vi "SetArrayDevParams.vi"(0 "Interface.lvclass":refnum<class "Interface.lvclass">, 1 "DescKword":string, 5 "Save":bool, 9 "Experiment.lvclass":refnum<class "Experiment.lvclass">, 11 "error in":errorcluster, 12 "ArrayFuncName":string) -> (3 "DataFileRef":refnum<file>, 4 "Interf.lvclass Out":refnum<class "Interface.lvclass">, 6 "DataFileName":path, 10 "Exp.lvclass Out":refnum<class "Experiment.lvclass">, 14 "Scan list":string[](array[string]), 15 "error out":errorcluster)   [LabVIEW 2019, in "Interface.lvclass"]
doc: "Ce Vi prend les données d'acquisition et les formatte en tableau de \"string\" pour ensuite les sauvegarder sous le format .txt"
uses:
  Interface.lvclass
  Experiment Class/Experiment.lvclass
  Interface.lvclass/Interface.ctl
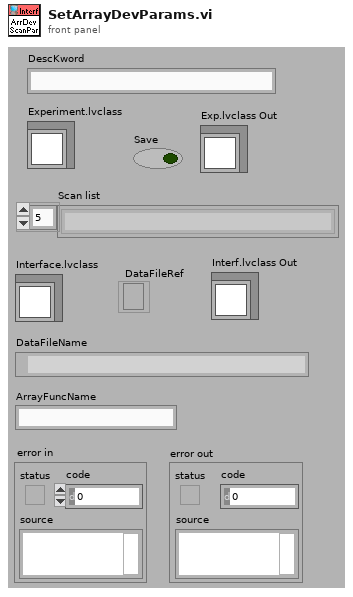
[diagram p1: front panel]
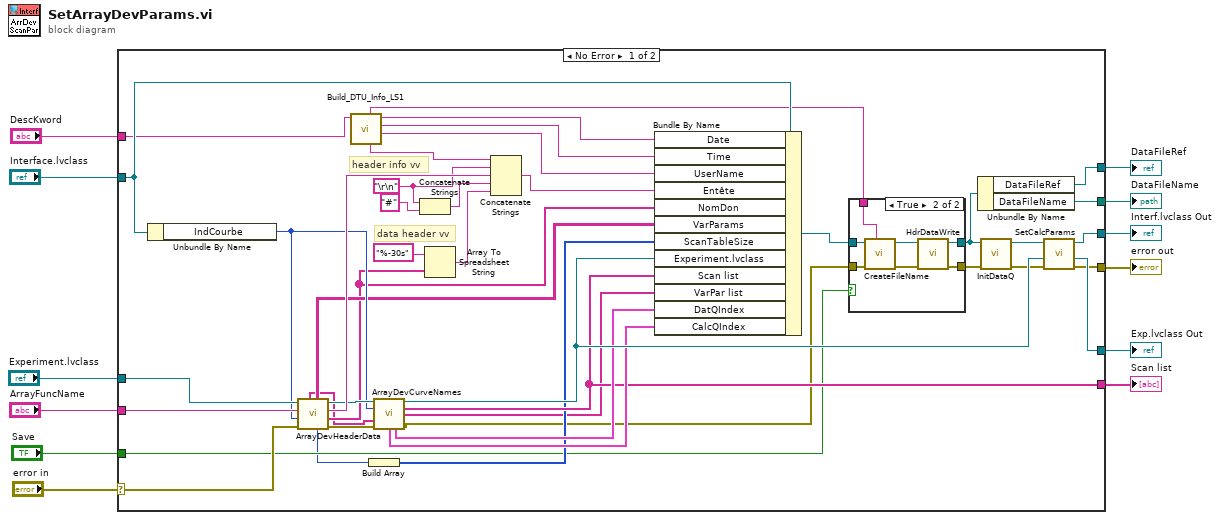
[diagram p0: block diagram]
diagram:
  n1 = case shown="No Error" "error in" {
    selector: "error in" -> [w31 w66]
    tunnel: [w42 w66] -> w12
    tunnel: [w45 w65] -> w9
    tunnel: "Interface.lvclass" -> [w39 w65]
    tunnel: [w50 _] -> w8
    tunnel: [w37 _] -> w7
    tunnel: [w47 _] -> w6
    tunnel: "Experiment.lvclass" -> [w46 w64]
    tunnel: [w43 w64] -> w4
    tunnel: "ArrayFuncName" -> [w38 _]
    tunnel: "Save" -> [w29 _]
    tunnel: "DescKword" -> [w15 _]
    frame No Error {
      w14 = "\r\n"
      # "data header vv"
      # "header info vv"
      n2 = Unbundle By Name(w39) -> ("IndCourbe"=w32:i64)
      n3 = call "ArrayDevHeaderData.vi"("error in"=w31, "IndCourbe"=w32, "ArrayFuncName"=w38, "Experiment.lvclass In"=w46) -> ("error out"=w52:errorcluster, "ArrNomDon"=w17:string[], "ArrHeaderPar"=w54:string, "Experiment.lvclass Out"=w53:refnum<class "Experiment.lvclass">, "Array Size"=w28:i32, "ArrVarParsOut"=w30:string[][], "ArrQdata"=w16:string[])  [unwired: 1 in]
      n4 = call "Build_DTU_Info_LS1.vi"("DescKword"=w15) -> ("ScanParUser"=w24:string, "ScanParTime"=w23:string, "ScanParDate"=w22:string, "DTU_HdrStr"=w26:string, "FileNmDTString"=w21:string)  [unwired: 4 in, 2 out]
      n5 = Build Array(w28) -> (w34:i32[])
      n6 = call "ArrayDevCurveNames.vi"("Experiment.lvclass In"=w53, "IndCourbe"=w32, "NomDon"=w16, "error in"=w52) -> ("Exp.lvclass Out"=w44:refnum<class "Experiment.lvclass">, "Scan list"=w37:string[], "VarPar list"=w19:string[], "CalcQIndex"=w40:cluster{"Tableau":i32[]}[], "DataQIndex"=w41:cluster{"Tableau":i32[]}[], "error out"=w20:errorcluster)  [unwired: 6 in]
      n7 = Concatenate Strings(w14, "#" ("chaîne")) -> (w27:string)
      n8 = Array To Spreadsheet String(array=w17, 3:"%-30s" ("format string")) -> (spreadsheet string=w48:string)  [unwired: 1 in]
      n9 = Concatenate Strings(w26, w14, w54, w27, w48) -> (w25:string)
      n10 = Bundle By Name(cluster=w39, "Date"=w22, "Time"=w23, "UserName"=w24, "Entête"=w25, "NomDon"=w17, "VarParams"=w30, "ScanTableSize"=w34, "Experiment.lvclass"=w44, "Scan list"=w37, "VarPar list"=w19, "DatQIndex"=w41, "CalcQIndex"=w40) -> (w51:refnum<class "Interface.lvclass">)
      n11 = case shown="True" w29 {
        tunnel: w51 -> [w55 w63]
        tunnel: w21 -> [_ w60]
        tunnel: [w55 w59] -> w18
        tunnel: [w56 w58] -> w36
        tunnel: w20 -> [w56 w57]
        frame False {
        }
        frame True {
          n12 = call "CreateFileName.vi"("Date"=w60, "error in (no error)"=w57, "Interface.lvclass"=w63) -> ("error out"=w61:errorcluster, "Interface.lvclass Out"=w62:refnum<class "Interface.lvclass">)  [unwired: 7 in]
          n13 = call "HdrDataWrite.vi"("error in (no error)"=w61, "Interface.lvclass"=w62) -> ("error out"=w58:errorcluster, "Interface.lvclassOut"=w59:refnum<class "Interface.lvclass">)  [unwired: 8 in]
        }
      }
      n14 = Unbundle By Name(w18) -> ("DataFileRef"=w47:refnum<file>, "DataFileName"=w50:path)
      n15 = call "InitDataQ.vi"("ErrorIn(No Error)"=w36, "Interface.lvclass"=w18) -> ("sortie d'erreur"=w35:errorcluster, "Interface.lvclass Out"=w33:refnum<class "Interface.lvclass">)  [unwired: 8 in]
      n16 = call "SetCalcParams.vi"("error in"=w35, "Experiment.lvclass"=w44, "Interface.lvclass"=w33) -> ("error out"=w42:errorcluster, "Experiment.lvclass Out"=w43:refnum<class "Experiment.lvclass">, "Interface.lvclass Out"=w45:refnum<class "Interface.lvclass">)  [unwired: 6 in]
    }
    frame Error {
    }
  }
  "error out" <- w12
  "Interf.lvclass Out" <- w9
  "DataFileName" <- w8
  "Scan list" <- w7
  "DataFileRef" <- w6
  "Exp.lvclass Out" <- w4
